vi "모터 조작.vi"() -> ()   [LabVIEW 2018]
uses:
  <vilib>/Instr/_visa.llb/VISA Configure Serial Port (Instr).vi
panel:
  in  "설정 변경":bool
  in  "현재 설정값 출력":bool
  in  "현재 위치를 0으로":bool
  in  "현재 위치 출력":bool
  in  "가속도":string
  in  "속도":string
  in  "위치":string
  out "에러 출력":errorcluster
  in  "정지":bool
  out "버퍼 읽기":string
  out "visa":T1
  in  "문자열":string
  in  "확인 버튼":bool
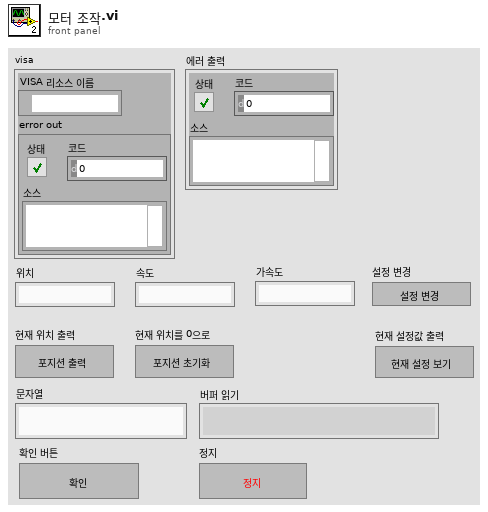
[diagram p1: front panel]
types:
  T1 = cluster{"VISA 리소스 이름":refnum<visa-resource-name>, "error out":errorcluster}
  T2 = cluster{"VISA resource name out":refnum<visa-resource-name>, "error out":errorcluster}
  T3 = typedef "모터용 컨트롤.ctl" = enum16{"초기화", "Idle", "정지", "설정출력", "포지션출력", "포지션초기화", "설정변경"}
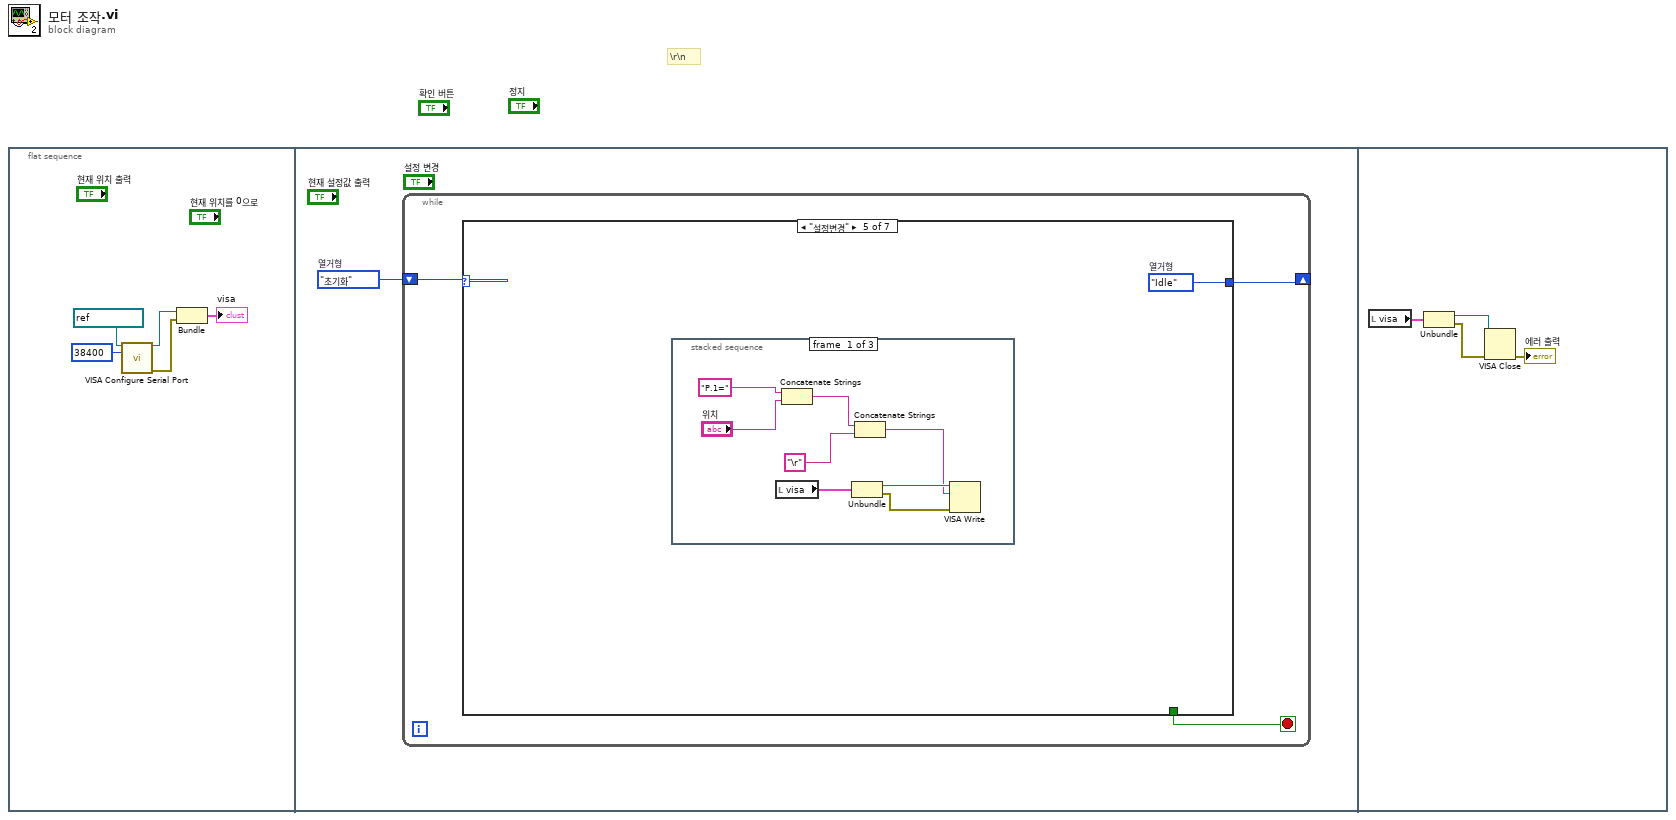
[diagram p0: block diagram]
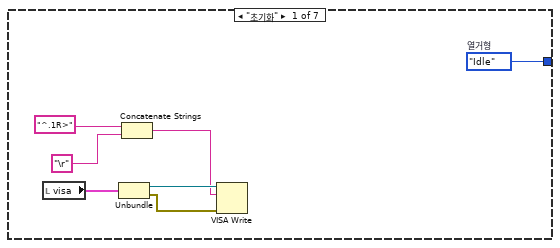
[diagram p2: hidden frame]
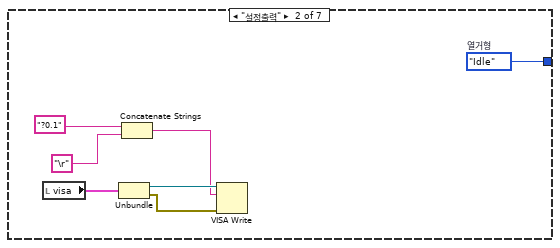
[diagram p3: hidden frame]
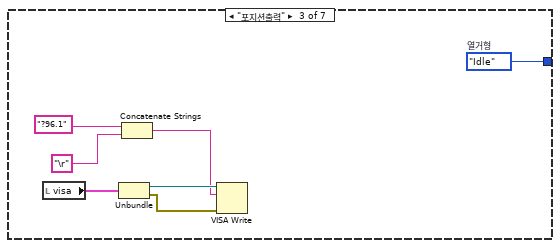
[diagram p4: hidden frame]
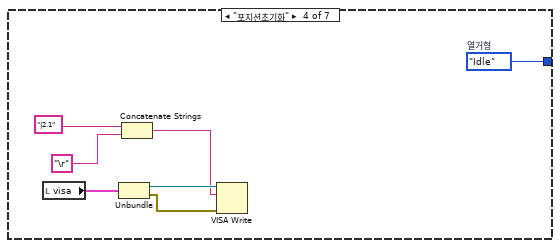
[diagram p5: hidden frame]
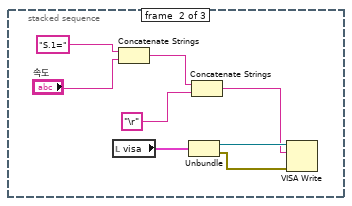
[diagram p6: hidden frame]
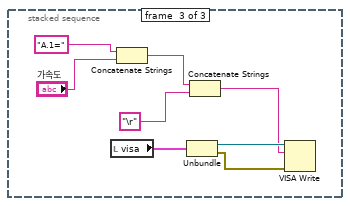
[diagram p7: hidden frame]
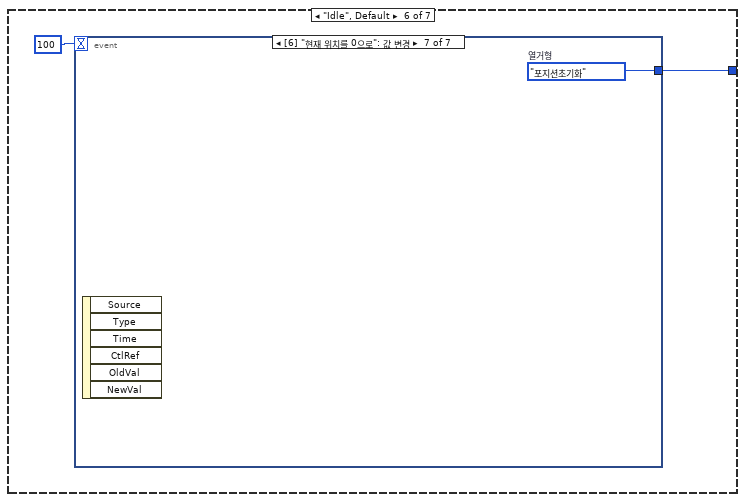
[diagram p8: hidden frame]
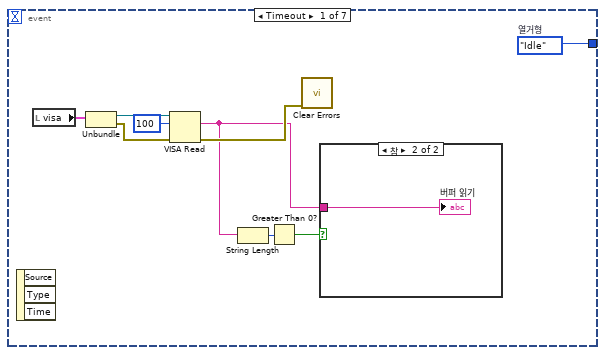
[diagram p9: hidden frame]
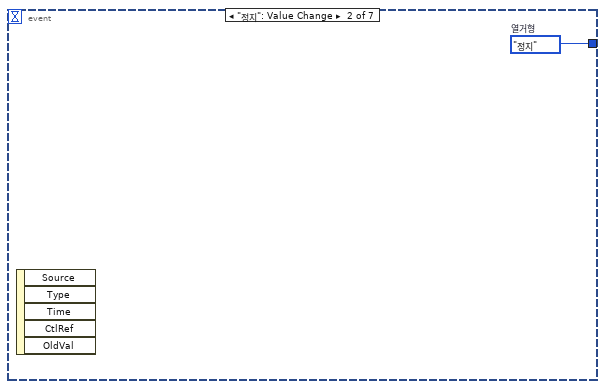
[diagram p11: hidden frame]
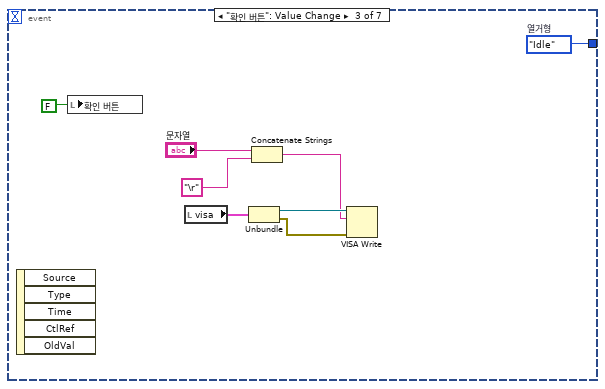
[diagram p12: hidden frame]
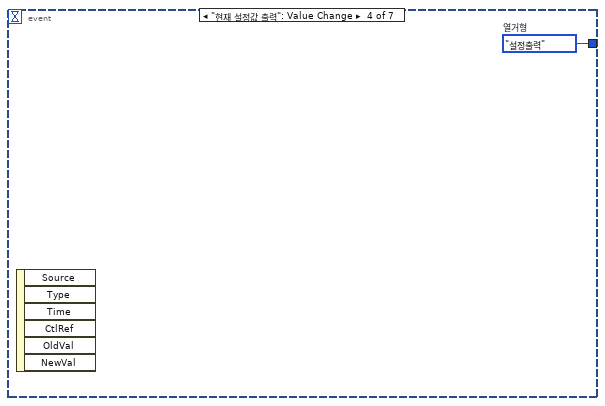
[diagram p13: hidden frame]
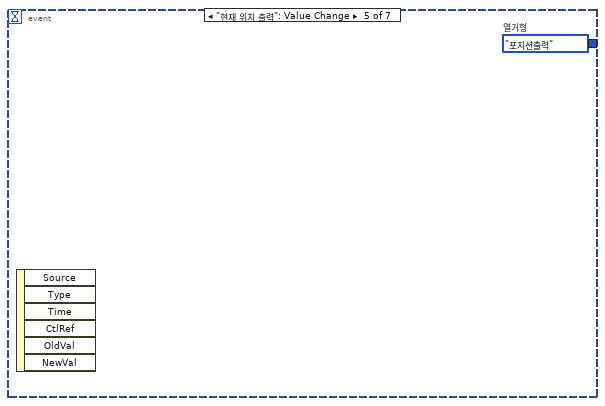
[diagram p14: hidden frame]
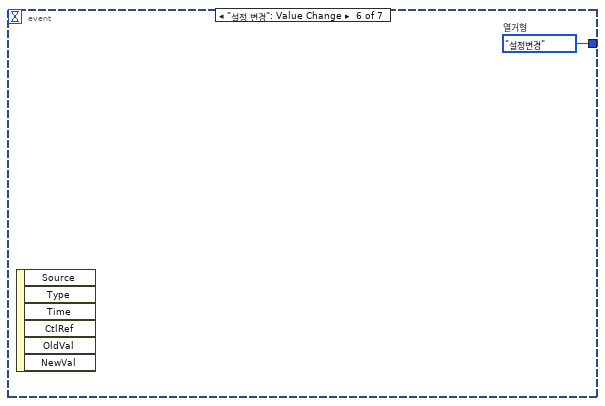
[diagram p15: hidden frame]
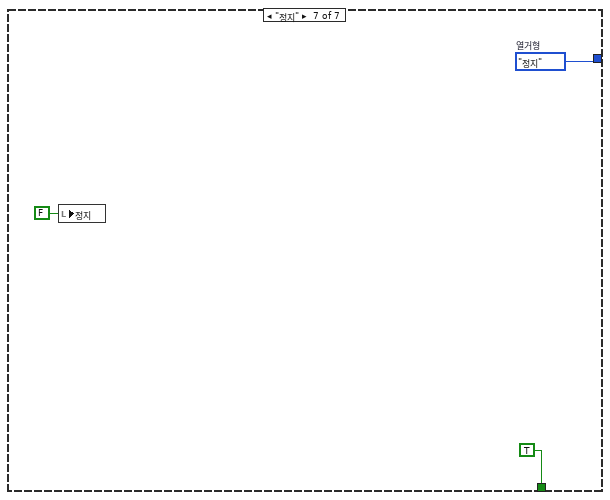
[diagram p16: hidden frame]
diagram:
  # "\\r\\n"
  n1 = flat-sequence {
    frame #0 {
      n2 = call-poly "VISA Configure Serial Port"("VISA resource name"=refnum<visa-resource-name> "COM19", "baud rate (9600)"=u32 38400) -> ("VISA resource name out"=w4:refnum<visa-resource-name>, "error out"=w3:errorcluster)  [unwired: 12 in]
      n3 = Bundle("VISA resource name out"=w4, "error out"=w3) -> (→"visa":T2)  [unwired: 1 in]
    }
    frame #1 {
      w6 = 모터용_컨트롤."초기화"  # 열거형
      n4 = while {
        shift-right: [w8] -> _
        shift-left: w6 -> [w9]
        stop <- w7 stop-if-true
        n5 = case shown="\"설정변경\"" w9 {
          tunnel: [w16 w23 w30 w37 w38 w63 w88] -> w8
          tunnel: [_ _ _ _ _ _ TRUE] -> w7
          frame "초기화" {
            w16 = 모터용_컨트롤."Idle"  # 열거형
            n6 = local read "visa"() -> (w10:T1)
            n7 = Unbundle(w10) -> ("VISA 리소스 이름"=w15:refnum<visa-resource-name>, "error out"=w14:errorcluster)
            n8 = Concatenate Strings("^.1R>", "\r" ("문자열")) -> (w12:string)
            n9 = VISA Write(VISA resource name=w15, write buffer=w12, error in (no error)=w14) -> ()  [unwired: 3 out]
          }
          frame "설정출력" {
            w23 = 모터용_컨트롤."Idle"  # 열거형
            n10 = local read "visa"() -> (w17:T1)
            n11 = Unbundle(w17) -> ("VISA 리소스 이름"=w22:refnum<visa-resource-name>, "error out"=w21:errorcluster)
            n12 = Concatenate Strings("?0.1", "\r" ("문자열")) -> (w19:string)
            n13 = VISA Write(VISA resource name=w22, write buffer=w19, error in (no error)=w21) -> ()  [unwired: 3 out]
          }
          frame "포지션출력" {
            w30 = 모터용_컨트롤."Idle"  # 열거형
            n14 = local read "visa"() -> (w24:T1)
            n15 = Unbundle(w24) -> ("VISA 리소스 이름"=w29:refnum<visa-resource-name>, "error out"=w28:errorcluster)
            n16 = Concatenate Strings("?96.1", "\r" ("문자열")) -> (w26:string)
            n17 = VISA Write(VISA resource name=w29, write buffer=w26, error in (no error)=w28) -> ()  [unwired: 3 out]
          }
          frame "포지션초기화" {
            w37 = 모터용_컨트롤."Idle"  # 열거형
            n18 = local read "visa"() -> (w31:T1)
            n19 = Unbundle(w31) -> ("VISA 리소스 이름"=w36:refnum<visa-resource-name>, "error out"=w35:errorcluster)
            n20 = Concatenate Strings("|2.1", "\r" ("문자열")) -> (w33:string)
            n21 = VISA Write(VISA resource name=w36, write buffer=w33, error in (no error)=w35) -> ()  [unwired: 3 out]
          }
          frame "설정변경" {
            w38 = 모터용_컨트롤."Idle"  # 열거형
            n22 = stacked-sequence {
              frame #0 {
                n23 = local read "visa"() -> (w42:T1)
                n24 = Concatenate Strings("P.1=", "위치") -> (w41:string)
                n25 = Unbundle(w42) -> ("VISA 리소스 이름"=w46:refnum<visa-resource-name>, "error out"=w45:errorcluster)
                n26 = Concatenate Strings(w41, "\r" ("문자열")) -> (w43:string)
                n27 = VISA Write(VISA resource name=w46, write buffer=w43, error in (no error)=w45) -> ()  [unwired: 3 out]
              }
              frame #1 {
                n28 = local read "visa"() -> (w50:T1)
                n29 = Concatenate Strings("S.1=", "속도") -> (w49:string)
                n30 = Unbundle(w50) -> ("VISA 리소스 이름"=w54:refnum<visa-resource-name>, "error out"=w53:errorcluster)
                n31 = Concatenate Strings(w49, "\r" ("문자열")) -> (w51:string)
                n32 = VISA Write(VISA resource name=w54, write buffer=w51, error in (no error)=w53) -> ()  [unwired: 3 out]
              }
              frame #2 {
                n33 = local read "visa"() -> (w58:T1)
                n34 = Concatenate Strings("A.1=", "가속도") -> (w57:string)
                n35 = Unbundle(w58) -> ("VISA 리소스 이름"=w62:refnum<visa-resource-name>, "error out"=w61:errorcluster)
                n36 = Concatenate Strings(w57, "\r" ("문자열")) -> (w59:string)
                n37 = VISA Write(VISA resource name=w62, write buffer=w59, error in (no error)=w61) -> ()  [unwired: 3 out]
              }
            }
          }
          frame "Idle", Default {
            n38 = event shown="[6] \"현재 위치를 0으로\": 값 변경" {
              selector: _ -> [_ _ _ _ _ _ _]
              dyn-events: _ -> [_ _ _ _ _ _ _]
              timeout: 100 -> [_ _ _ _ _ _ _]
              tunnel: [w65 w75 w76 w84 w85 w86 w87] -> w63
              event Timeout {
                w65 = 모터용_컨트롤."Idle"  # 열거형
                n39 = event-data() -> ()  [unwired: 1 in, 3 out]
                n40 = local read "visa"() -> (w73:T1)
                n41 = Unbundle(w73) -> ("VISA 리소스 이름"=w72:refnum<visa-resource-name>, "error out"=w71:errorcluster)
                n42 = VISA Read(VISA resource name=w72, byte count=u32 100 ("바이트 카운트"), error in (no error)=w71) -> (read buffer=w68:string, error out=w69:errorcluster)  [unwired: 2 out]
                n43 = String Length(string=w68) -> (length=w67:i32)
                n44 = Greater Than 0?(x=w67) -> (x > 0?=w66:bool)
                n45 = call <vilib>:"Clear Errors.vi"("error in (no error)"=w69) -> ()  [unwired: 5 in, 2 out]
                n46 = case shown="참" w66 {
                  tunnel: w68 -> [_ w74]
                  frame False {
                  }
                  frame True {
                    "버퍼 읽기" <- w74
                  }
                }
              }
              event "정지": Value Change {
                w75 = 모터용_컨트롤."정지"  # 열거형
                n47 = event-data() -> ()  [unwired: 1 in, 5 out]
              }
              event "확인 버튼": Value Change {
                w76 = 모터용_컨트롤."Idle"  # 열거형
                n48 = event-data() -> ()  [unwired: 1 in, 5 out]
                n49 = local write "확인 버튼"(FALSE ("확인 버튼")) -> ()
                n50 = local read "visa"() -> (w82:T1)
                n51 = Unbundle(w82) -> ("VISA 리소스 이름"=w81:refnum<visa-resource-name>, "error out"=w80:errorcluster)
                n52 = Concatenate Strings("문자열", "\r" ("문자열")) -> (w78:string)
                n53 = VISA Write(VISA resource name=w81, write buffer=w78, error in (no error)=w80) -> ()  [unwired: 3 out]
              }
              event "현재 설정값 출력": Value Change {
                w84 = 모터용_컨트롤."설정출력"  # 열거형
                n54 = event-data() -> ()  [unwired: 1 in, 6 out]
              }
              event "현재 위치 출력": Value Change {
                w85 = 모터용_컨트롤."포지션출력"  # 열거형
                n55 = event-data() -> ()  [unwired: 1 in, 6 out]
              }
              event "설정 변경": Value Change {
                w86 = 모터용_컨트롤."설정변경"  # 열거형
                n56 = event-data() -> ()  [unwired: 1 in, 6 out]
              }
              event "현재 위치를 0으로": Value Change {
                w87 = 모터용_컨트롤."포지션초기화"  # 열거형
                n57 = event-data() -> ()  [unwired: 1 in, 6 out]
              }
            }
          }
          frame "정지" {
            w88 = 모터용_컨트롤."정지"  # 열거형
            n58 = local write "정지"(FALSE ("정지")) -> ()
          }
        }
      }
    }
    frame #2 {
      n59 = local read "visa"() -> (w94:T1)
      n60 = Unbundle(w94) -> ("VISA 리소스 이름"=w93:refnum<visa-resource-name>, "error out"=w92:errorcluster)
      n61 = VISA Close(VISA resource name=w93, error in (no error)=w92) -> (error out=→"에러 출력":errorcluster)
    }
  }
